vi "solar Interlocks.vi"(8 "error in (no error)":errorcluster, 9 "DATA in":variant, 10 "MSG in":string, 11 "solar in":refnum<class "solar.lvclass">) -> (0 "error out":errorcluster, 1 "DATA out":variant, 2 "MSG out":string, 3 "solar out":refnum<class "solar.lvclass">)   [LabVIEW 2018, in "solar.lvclass"]
doc: "Handle target interlock checks."
uses:
  solar.lvclass
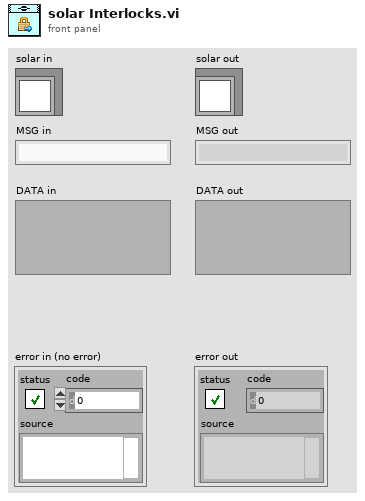
[diagram p1: front panel]
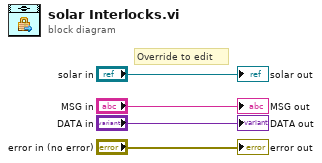
[diagram p0: block diagram]
diagram:
  # "Override to edit"
  "error out" <- "error in (no error)"
  "solar out" <- "solar in"
  "MSG out" <- "MSG in"
  "DATA out" <- "DATA in"
